vi "Write configuration.vi"(8 "error in (no error)":errorcluster, 11 "Thorcam in":refnum<class "Thorcam.lvclass">) -> (0 "error out":errorcluster, 3 "Thorcam out":refnum<class "Thorcam.lvclass">)   [LabVIEW 2012, in "Thorcam.lvclass"]
doc: "Writes the configuration cluster into the configuration file. Configuration file is XML-based. It's name is <component ID>.xml"
uses:
  Thorcam.lvclass
  <vilib>/Distrio/Murmex/Murmex/Murmex.lvclass
  Thorcam.lvclass/Thorcam.ctl
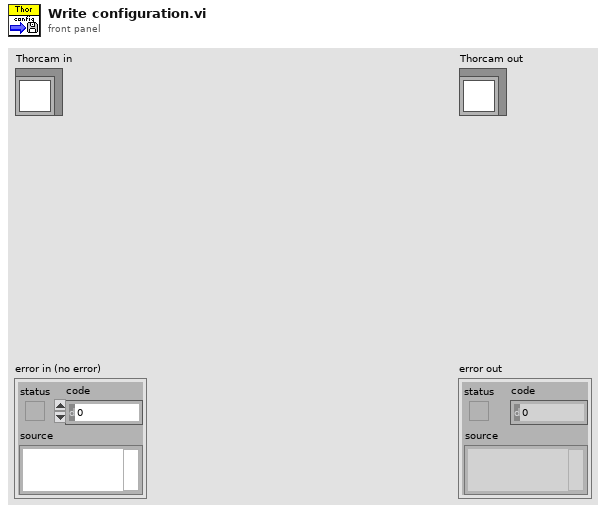
[diagram p1: front panel]
types:
  T1 = typedef "Thorcam.lvclass/configuration.ctl" = cluster{"camera ID":u32, "Settings":string}
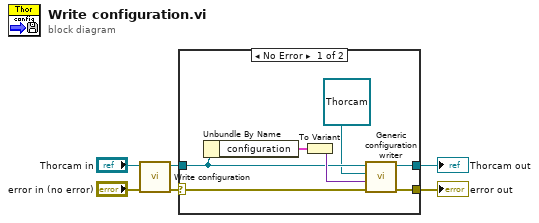
[diagram p0: block diagram]
diagram:
  n1 = call-parent "Write configuration.vi"("error in (no error)"="error in (no error)", "Murmex in"="Thorcam in") -> ("error out"=w4:errorcluster, "Murmex out"=w3:refnum<class "Thorcam.lvclass">)  [unwired: 8 in]
  n2 = case shown="No Error" w4 {
    selector: w4 -> [w11 w14]
    tunnel: w3 -> [w10 w15]
    tunnel: [w8 w15] -> w2
    tunnel: [w7 w14] -> w1
    frame No Error {
      n3 = Unbundle By Name(w10) -> ("configuration"=w12:T1)
      n4 = To Variant(anything=w12) -> (Variant=w13:variant)
      n5 = call <vilib>:"Generic configuration writer.vi"("error in (no error)"=w11, "configuration"=w13, "inheritance level"=refnum<class "Thorcam.lvclass"> refnum ("Thorcam"), "MurmexBase in"=w10) -> ("error out"=w7:errorcluster, "MurmexBase out"=w8:refnum<class "Thorcam.lvclass">)  [unwired: 6 in]
    }
    frame Error {
    }
  }
  "error out" <- w1
  "Thorcam out" <- w2
